vi "GT Set Laser Dis Mode.vi"(0 "cardNum":i16, 1 "pScale":dbl, 5 "mode":i16, 7 "source":i16, 9 "pPos":i32, 11 "error in (no error)":errorcluster caption="错误输入（无错误）", 12 "channel":i16) -> (3 "pScale out":dbl, 4 "function return":i16, 10 "pPos out":i32, 15 "error out":errorcluster caption="错误输出")   [LabVIEW 2014, in "gts.lvlib"]
doc: "GT_API GT_SetLaserDisMode(short cardNum,short mode,short source,long *pPos,double *pScale,short channel=0);"
uses:
  gts.lvlib
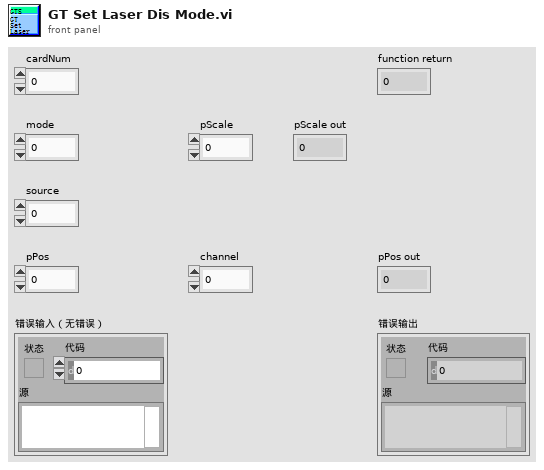
[diagram p1: front panel]
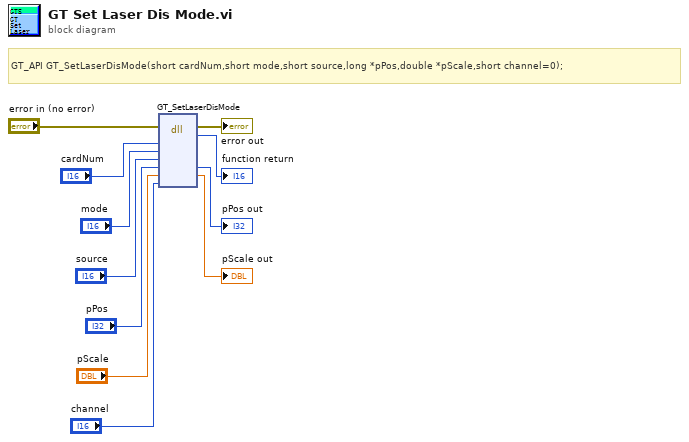
[diagram p0: block diagram]
diagram:
  # "GT_API GT_SetLaserDisMode(short cardNum,short mode,short source,long *pPos,double *pScale,short channel=0);"
  n1 = dll-call lib="PTH2habs D固高科技资料GTS控制卡GTS卡18年上半年资料dllVC32bit\nmulti_cardgts.*" fn="GT_SetLaserDisMode"(error in="error in (no error)", "cardNum"="cardNum", "mode"="mode", "source"="source", "pPos"="pPos", "pScale"="pScale", "channel"="channel") -> (error out=→"error out":errorcluster, →"function return":i16, "pPos"=→"pPos out":i32, "pScale"=→"pScale out":dbl)  [unwired: 6 in, 1 out]
